vi "Read BRAND SELECTED CY.vi"(8 "error in (no error)":errorcluster, 11 "TI in":refnum<class "CYPRESS.lvclass">) -> (0 "error out":errorcluster, 2 "BRAND SELECTED":enum16{"NXP", "CYPRESS", "SIMULATED"}(ring), 3 "TI out":refnum<class "CYPRESS.lvclass">)   [LabVIEW 2019, in "CYPRESS.lvclass"]
uses:
  CYPRESS.lvclass
  CYPRESS.lvclass/CYPRESS.ctl
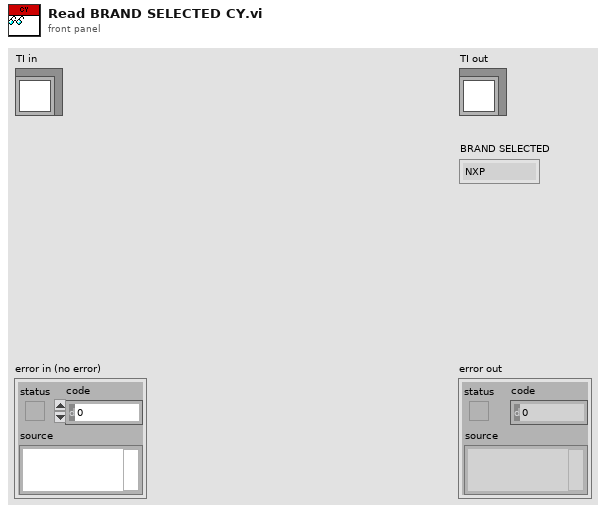
[diagram p1: front panel]
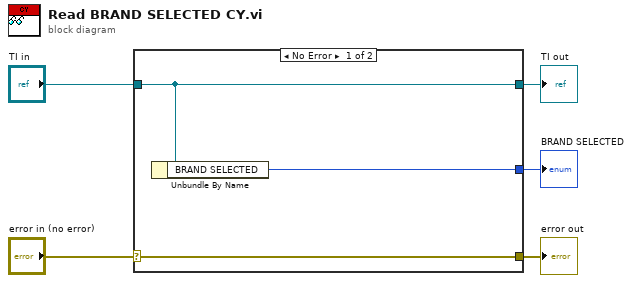
[diagram p0: block diagram]
diagram:
  n1 = case shown="No Error" "error in (no error)" {
    selector: "error in (no error)" -> [w8 w9]
    tunnel: [w8 w9] -> w4
    tunnel: [w7 w10] -> w2
    tunnel: "TI in" -> [w7 w10]
    tunnel: [w6 _] -> w1
    frame No Error {
      n2 = Unbundle By Name(w7) -> ("BRAND SELECTED"=w6:enum16{"NXP", "CYPRESS", "SIMULATED"})
    }
    frame Error {
    }
  }
  "error out" <- w4
  "TI out" <- w2
  "BRAND SELECTED" <- w1
